vi "Configure Trigger.vi"(8 "error in (no error)":errorcluster, 9 "Mode":T1=enum."FALLING", 11 "VISA resource name":refnum<visa-resource-name>) -> (0 "error out":errorcluster, 3 "VISA resource name out":refnum<visa-resource-name>)   [LabVIEW 2020, in "BDAQ-6104.lvlib"]
uses:
  <instrlib>/BDAQ-6104/BDAQ-6104.lvlib
  <instrlib>/BDAQ-6104/Private/Edge Triger Type.ctl
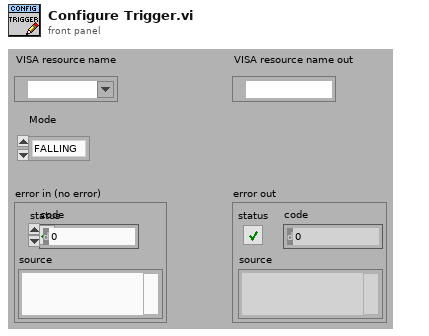
[diagram p1: front panel]
types:
  T1 = typedef "BDAQ-6104.lvlib/Edge Triger Type.ctl" = enum16{"CHANGE", "FALLING", "RISING"}
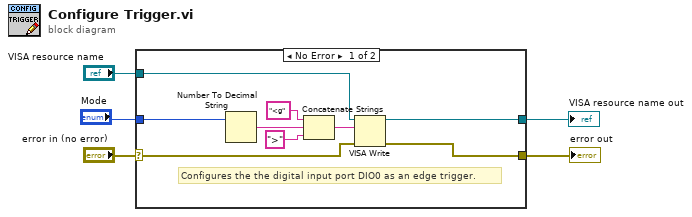
[diagram p0: block diagram]
diagram:
  n1 = case shown="No Error" "error in (no error)" {
    selector: "error in (no error)" -> [w7 w15]
    tunnel: "VISA resource name" -> [w14 w16]
    tunnel: [w9 w15] -> w4
    tunnel: [w8 w16] -> w3
    tunnel: "Mode" -> [w6 _]
    frame No Error {
      # "Configures the the digital input port DIO0 as an edge trigger."
      n2 = Number To Decimal String(number=w6) -> (decimal integer string=w12:string)  [unwired: 1 in]
      n3 = Concatenate Strings("<g", w12, ">") -> (w10:string)
      n4 = VISA Write(VISA resource name=w14, write buffer=w10, error in (no error)=w7) -> (VISA resource name out=w8:refnum<visa-resource-name>, error out=w9:errorcluster)  [unwired: 1 out]
    }
    frame Error {
    }
  }
  "error out" <- w4
  "VISA resource name out" <- w3
